vi "Calculate Stitching Data.vi"(8 "error in":errorcluster, 11 "Physical Images in":T1[](array[typedef])) -> (0 "error out":errorcluster, 1 "Image overlay positions":cluster{i32, i32}[](array[cluster]), 2 "Image Rescale Resolutions":cluster{"Cols":i32, "Rows":i32}[](array[cluster]), 3 "Target Resolution":cluster{"cols":i32, "rows":i32}, 4 "Target FOV":cluster{"x(mm)":dbl, "y(mm)":dbl}, 5 "Target Center":refnum<class "Vec3d Class.lvclass">)   [LabVIEW 2017]
uses:
  Type Definitions/Physical Image.ctl
  Vec3d Class/Vec3d Class.lvclass
  <vilib>/vision/Image Controls.llb/IMAQ Image.ctl
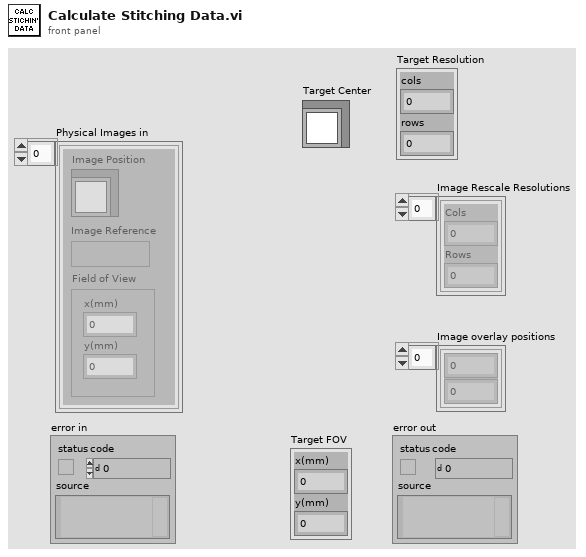
[diagram p1: front panel]
types:
  T1 = typedef "Physical Image.ctl" = cluster{"Image Position":refnum<class "Vec3d Class.lvclass">, "Image Reference":T2, "Field of View":cluster{"x(mm)":dbl, "y(mm)":dbl}}
  T2 = typedef "IMAQ Image.ctl" = refnum<image>
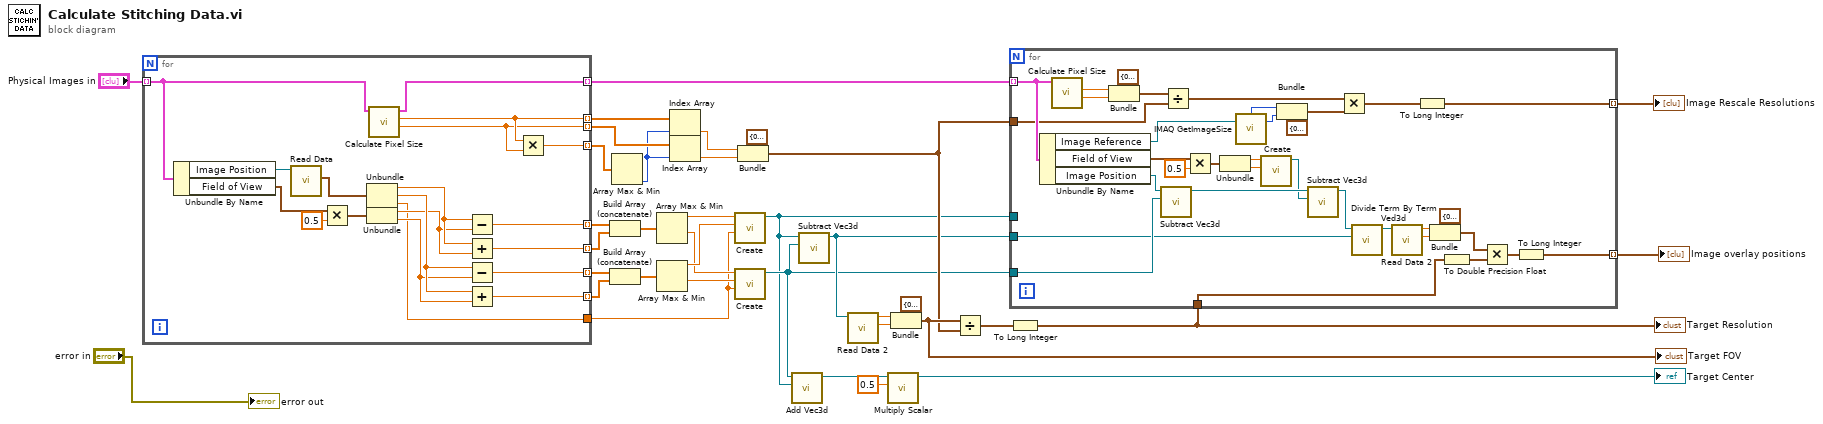
[diagram p0: block diagram]
diagram:
  n1 = for {
    tunnel: "Physical Images in" -> [w54] mode=indexing
    tunnel: [w53] -> w20 mode=indexing
    tunnel: [w52] -> w34 mode=indexing
    tunnel: [w51] -> w33 mode=indexing
    tunnel: [w50] -> w35 mode=indexing
    tunnel: [w41] -> w31 mode=indexing
    tunnel: [w40] -> w27 mode=indexing
    tunnel: [w39] -> w30 mode=indexing
    tunnel: [w38] -> w28 mode=indexing
    tunnel: [w37] -> w21
    n2 = Unbundle By Name(w54) -> ("Image Position"=w55:refnum<class "Vec3d Class.lvclass">, "Field of View"=w48:cluster{"x(mm)":dbl, "y(mm)":dbl})
    n3 = call-dynamic "Read Data.vi"("Vec3d Class in"=w55) -> ("Data"=w49:cluster{"X":dbl, "Y":dbl, "Z":dbl})  [unwired: 8 in, 2 out]
    n4 = Multiply(x=w48, y=0.5) -> (x*y=w46:cluster{"x(mm)":dbl, "y(mm)":dbl})
    n5 = Unbundle(w49) -> ("X"=w45:dbl, "Y"=w44:dbl, "Z"=w37:dbl)
    n6 = Unbundle(w46) -> ("x(mm)"=w43:dbl, "y(mm)"=w42:dbl)
    n7 = call "Calculate Pixel Size.vi"("Physical Image in"=w54) -> ("Pixel Size y(mm)"=w51:dbl, "Pixel Size x(mm)"=w52:dbl, "Physical Image Out"=w53:T1)  [unwired: 7 in, 1 out]
    n8 = Subtract(x=w45, y=w43) -> (x-y=w41:dbl)
    n9 = Add(x=w45, y=w43) -> (x+y=w39:dbl)
    n10 = Subtract(x=w44, y=w42) -> (x-y=w40:dbl)
    n11 = Add(x=w44, y=w42) -> (x+y=w38:dbl)
    n12 = Multiply(x=w52, y=w51) -> (x*y=w50:dbl)
  }
  n13 = Build Array (concatenate)(w31, w30) -> (w29:dbl[])
  n14 = Build Array (concatenate)(w27, w28) -> (w26:dbl[])
  n15 = Array Max & Min(array=w35) -> (min index (indices)=w32:i32)  [unwired: 3 out]
  n16 = Array Max & Min(array=w29) -> (max value=w25:dbl, min value=w23:dbl)  [unwired: 2 out]
  n17 = Array Max & Min(array=w26) -> (max value=w24:dbl, min value=w22:dbl)  [unwired: 2 out]
  n18 = Index Array(array=w34, index=w32) -> (element=w18:dbl)
  n19 = Index Array(array=w33, index=w32) -> (element=w17:dbl)
  n20 = call "Create.vi"("Z"=w21, "Y"=w24, "X"=w25) -> ("Vec3d Class out"=w4:refnum<class "Vec3d Class.lvclass">)  [unwired: 7 in, 1 out]
  n21 = call "Create.vi"("Z"=w21, "Y"=w22, "X"=w23) -> ("Vec3d Class out"=w5:refnum<class "Vec3d Class.lvclass">)  [unwired: 7 in, 1 out]
  n22 = Bundle(cluster=cluster{"x(mm)":dbl, "y(mm)":dbl} {"x(mm)"=0.0, "y(mm)"=0.0} ("x*y"), "x(mm)"=w18, "y(mm)"=w17) -> (w12:cluster{"x(mm)":dbl, "y(mm)":dbl})
  n23 = call-dynamic "Add Vec3d.vi"(10:"Vec3d Class in"=w4, 11:"Vec3d Class in"=w5) -> ("Vec3d Class out"=w3:refnum<class "Vec3d Class.lvclass">)  [unwired: 8 in, 1 out]
  n24 = call "Subtract Vec3d.vi"("Vec3d in 2"=w5, "Vec3d in 1"=w4) -> ("Vec3d Class out"=w10:refnum<class "Vec3d Class.lvclass">)  [unwired: 8 in, 1 out]
  n25 = call-dynamic "Read Data 2.vi"("Vec3d in"=w10) -> ("Y"=w14:dbl, "X"=w15:dbl)  [unwired: 7 in, 2 out]
  n26 = call-dynamic "Multiply Scalar.vi"("Scale"=0.5, "Vec3d in"=w3) -> ("Vec3d out"=→"Target Center":refnum<class "Vec3d Class.lvclass">)  [unwired: 8 in, 1 out]
  n27 = Bundle(cluster=cluster{"x(mm)":dbl, "y(mm)":dbl} {"x(mm)"=0.0, "y(mm)"=0.0} ("x*y"), "x(mm)"=w15, "y(mm)"=w14) -> (w13:cluster{"x(mm)":dbl, "y(mm)":dbl})
  "Target FOV" <- w13
  n28 = Divide(x=w13, y=w12) -> (x/y=w11:cluster{"x(mm)":dbl, "y(mm)":dbl})
  n29 = To Long Integer(number=w11) -> (32bit integer=w9:cluster{"x(mm)":i32, "y(mm)":i32})
  "Target Resolution" <- w9
  n30 = for {
    tunnel: w20 -> [w88] mode=indexing
    tunnel: w12 -> [w63]
    tunnel: w4 -> [_]
    tunnel: w5 -> [w86]
    tunnel: w10 -> [w85]
    tunnel: w9 -> [w70]
    tunnel: [w71] -> w8 mode=indexing
    tunnel: [w56] -> w7 mode=indexing
    (unwired) cluster{"x(mm)":dbl, "y(mm)":dbl} {"x(mm)"=0.0, "y(mm)"=0.0} ("x*y")
    n31 = Unbundle By Name(w88) -> ("Image Reference"=w68:T2, "Field of View"=w83:cluster{"x(mm)":dbl, "y(mm)":dbl}, "Image Position"=w87:refnum<class "Vec3d Class.lvclass">)
    n32 = call "Calculate Pixel Size.vi"("Physical Image in"=w88) -> ("Pixel Size y(mm)"=w65:dbl, "Pixel Size x(mm)"=w66:dbl)  [unwired: 7 in, 2 out]
    n33 = Bundle(cluster=cluster{"x(mm)":dbl, "y(mm)":dbl} {"x(mm)"=0.0, "y(mm)"=0.0} ("x*y"), "x(mm)"=w66, "y(mm)"=w65) -> (w64:cluster{"x(mm)":dbl, "y(mm)":dbl})
    n34 = call "Subtract Vec3d.vi"("Vec3d in 2"=w86, "Vec3d in 1"=w87) -> ("Vec3d Class out"=w79:refnum<class "Vec3d Class.lvclass">)  [unwired: 8 in, 1 out]
    n35 = Divide(x=w64, y=w63) -> (x/y=w59:cluster{"x(mm)":dbl, "y(mm)":dbl})
    n36 = Multiply(x=w83, y=0.5) -> (x*y=w82:cluster{"x(mm)":dbl, "y(mm)":dbl})
    n37 = Unbundle(w82) -> ("x(mm)"=w81:dbl, "y(mm)"=w80:dbl)
    n38 = call "IMAQ GetImageSize"("Image"=w68) -> ("Y Resolution"=w60:i32, "X Resolution"=w61:i32)  [unwired: 3 in, 1 out]
    n39 = call "Create.vi"("Y"=w80, "X"=w81) -> ("Vec3d Class out"=w78:refnum<class "Vec3d Class.lvclass">)  [unwired: 8 in, 1 out]
    n40 = Bundle(cluster=cluster{"x(mm)":dbl, "y(mm)":dbl} {"x(mm)"=0.0, "y(mm)"=0.0} ("x*y"), "x(mm)"=w61, "y(mm)"=w60) -> (w58:cluster{"x(mm)":dbl, "y(mm)":dbl})
    n41 = call "Subtract Vec3d.vi"("Vec3d in 2"=w78, "Vec3d in 1"=w79) -> ("Vec3d Class out"=w77:refnum<class "Vec3d Class.lvclass">)  [unwired: 8 in, 1 out]
    n42 = Multiply(x=w59, y=w58) -> (x*y=w57:cluster{"x(mm)":dbl, "y(mm)":dbl})
    n43 = call-dynamic "Divide Term By Term Ved3d.vi"("Vec3d in 2"=w85, "Vec3d in 1"=w77) -> ("Vec3d Class out"=w74:refnum<class "Vec3d Class.lvclass">)  [unwired: 8 in, 1 out]
    n44 = call-dynamic "Read Data 2.vi"("Vec3d in"=w74) -> ("Y"=w75:dbl, "X"=w76:dbl)  [unwired: 7 in, 2 out]
    n45 = To Long Integer(number=w57) -> (32bit integer=w56:cluster{"x(mm)":i32, "y(mm)":i32})
    n46 = Bundle("X"=w76, "Y"=w75) -> (w73:cluster{"X":dbl, "Y":dbl})  [unwired: 1 in]
    n47 = To Double Precision Float(number=w70) -> (double precision float=w69:cluster{"x(mm)":dbl, "y(mm)":dbl})
    n48 = Multiply(x=w73, y=w69) -> (x*y=w72:cluster{dbl, dbl})
    n49 = To Long Integer(number=w72) -> (32bit integer=w71:cluster{i32, i32})
  }
  "Image Rescale Resolutions" <- w7
  "Image overlay positions" <- w8
  "error out" <- "error in"
